vi "find timing tag indices.vi"(8 "error in":errorcluster, 10 "timing reporting":T1, 11 "data dictionary in":refnum<class "data dictionary.lvclass">) -> (0 "error out":errorcluster, 1 "dt ns":i32, 2 "late count":i32, 3 "late boolean":i32)   [LabVIEW 2013, in "Standard Engine Runtime.lvclass"]
uses:
  Standard Engine Runtime.lvclass
  <vilib>/NI/Tag Bus/dictionary/data dictionary.lvclass
  Configuration/timing reporting tags.ctl
  <vilib>/NI/Tag Bus/dictionary/data dictionary.lvclass/data dictionary.ctl
  <vilib>/NI/Tag Bus/dictionary/lookup polymorphs/locate Boolean.vi
  <vilib>/NI/Tag Bus/dictionary/lookup polymorphs/locate U32.vi
  <vilib>/NI/Tag Bus/dictionary/lookup polymorphs/locate U64.vi
  <vilib>/NI/Tag Bus/dictionary/search/find data index.vi
  <vilib>/NI/Tag Bus/dictionary/search/search string list.vi
  <vilib>/NI/Tag Bus/dictionary/tag not found.vi
  Configuration/Standard Engine Configuration.lvclass
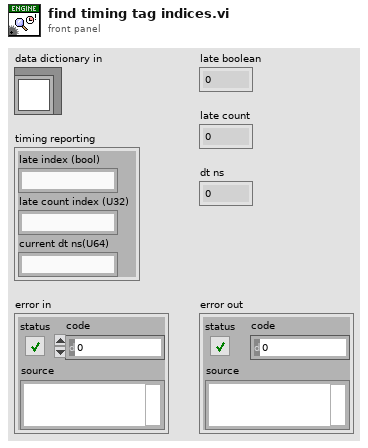
[diagram p1: front panel]
types:
  T1 = typedef "Standard Engine Configuration.lvclass/timing reporting tags.ctl" = cluster{"late index (bool)":string, "late count index (U32)":string, "current dt ns(U64)":string}
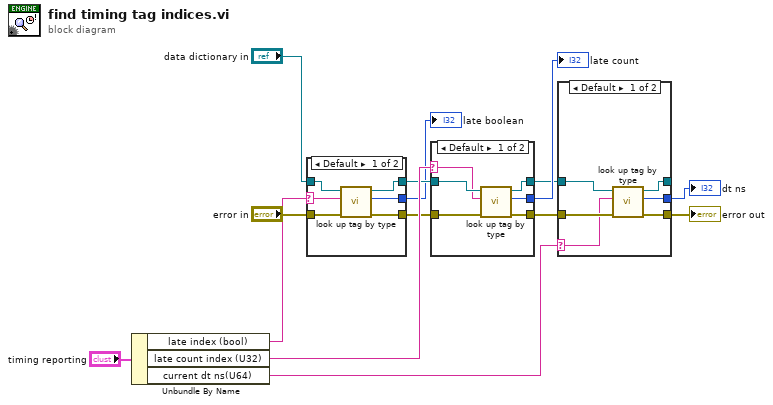
[diagram p0: block diagram]
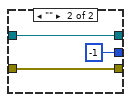
[diagram p2: hidden frame]
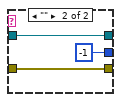
[diagram p3: hidden frame]
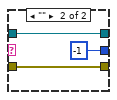
[diagram p4: hidden frame]
diagram:
  n1 = Unbundle By Name("timing reporting") -> ("late index (bool)"=w2:string, "late count index (U32)"=w10:string, "current dt ns(U64)"=w12:string)
  n2 = case shown="Default" w2 {
    selector: w2 -> [w16 _]
    tunnel: [w19 w23] -> w9
    tunnel: "error in" -> [w20 w23]
    tunnel: "data dictionary in" -> [w17 w22]
    tunnel: [w18 w22] -> w8
    tunnel: [w15 -1] -> w5
    frame Default {
      n3 = call-poly <vilib>:"look up tag by type.vi"("error in"=w20, "name"=w16, "data dictionary in"=w17) -> ("error out"=w19:errorcluster, "index"=w15:i32, "data dictionary out"=w18:refnum<class "data dictionary.lvclass">)  [unwired: 6 in]
    }
    frame "" {
    }
  }
  "late boolean" <- w5
  n4 = case shown="Default" w10 {
    selector: w10 -> [w25 _]
    tunnel: [w28 w32] -> w11
    tunnel: w9 -> [w29 w32]
    tunnel: w8 -> [w26 w31]
    tunnel: [w27 w31] -> w7
    tunnel: [w24 -1] -> w14
    frame Default {
      n5 = call-poly <vilib>:"look up tag by type.vi"("error in"=w29, "name"=w25, "data dictionary in"=w26) -> ("error out"=w28:errorcluster, "index"=w24:i32, "data dictionary out"=w27:refnum<class "data dictionary.lvclass">)  [unwired: 6 in]
    }
    frame "" {
    }
  }
  "late count" <- w14
  n6 = case shown="Default" w12 {
    selector: w12 -> [w34 _]
    tunnel: [w37 w41] -> w6
    tunnel: w11 -> [w38 w41]
    tunnel: w7 -> [w35 w40]
    tunnel: [w36 w40] -> _
    tunnel: [w33 -1] -> w13
    frame Default {
      n7 = call-poly <vilib>:"look up tag by type.vi"("error in"=w38, "name"=w34, "data dictionary in"=w35) -> ("error out"=w37:errorcluster, "index"=w33:i32, "data dictionary out"=w36:refnum<class "data dictionary.lvclass">)  [unwired: 6 in]
    }
    frame "" {
    }
  }
  "dt ns" <- w13
  "error out" <- w6
